vi "SeCrTs-Datalog Redundant NS creater.vi"(9 "Data FIFO Ref":T1, 11 "Queue in":refnum<queue>) -> ()   [LabVIEW 2022 SP3]
uses:
  RT Controls/SeCrTs-Data FIFO.ctl
  RT Controls/SeCrTs-DiplayPC comm ctrl.ctl
  SeCrTs-RT_Global_R.vi
  <resource>/objmgr/ni.dex.rc
panel:
  out "Numeric":i32
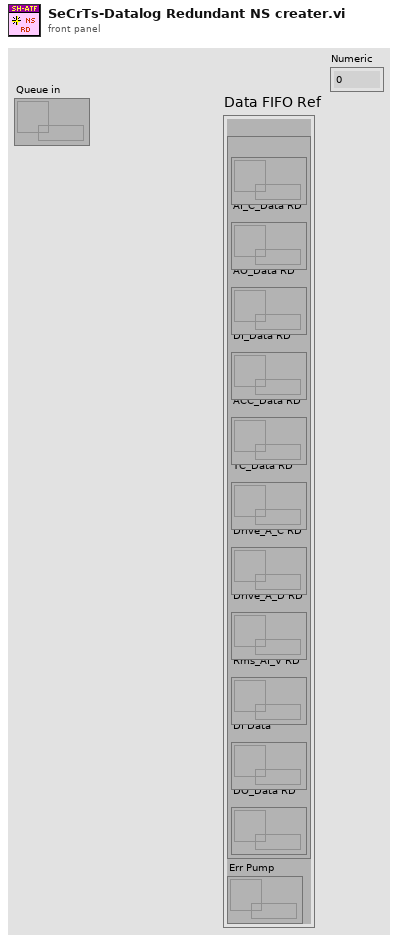
[diagram p1: front panel]
types:
  T1 = typedef "SeCrTs-Data FIFO.ctl" = cluster{"RD":cluster{"AI_V_Data RD":refnum<queue>, "AI_C_Data RD":refnum<queue>, "AO_Data RD":refnum<queue>, "DI_Data RD":refnum<queue>, "ACC_Data RD":refnum<queue>, "TC_Data RD":refnum<queue>, "Drive_A_C RD":refnum<queue>, "Drive_A_D RD":refnum<queue>, "Rms_AI_V RD":refnum<queue>, "DI Data":refnum<queue>, "DO_Data RD":refnum<queue>}, "Err Pump":refnum<queue>}
  T2 = typedef "SeCrTs-DiplayPC comm ctrl.ctl" = enum16{"Initialize", "Listen for UI Writer", "Send RT Data"}
  T3 = cluster{"Start DAQ":bool, "Stop DAQ":bool, "RT Stop":bool, "RT Exit":bool, "Start Seq":bool}
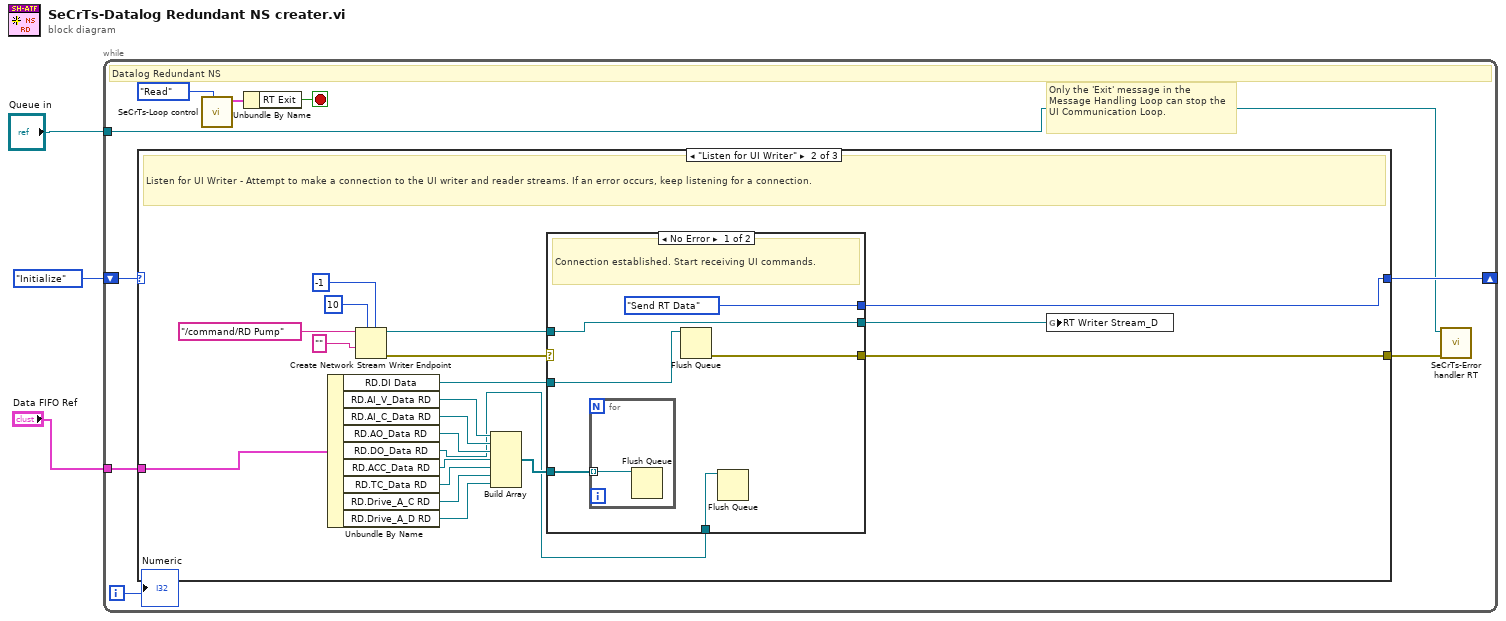
[diagram p0: block diagram]
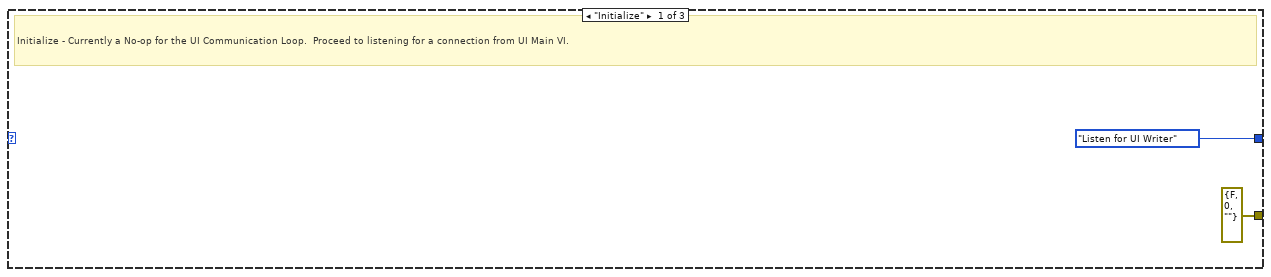
[diagram p2: hidden frame]
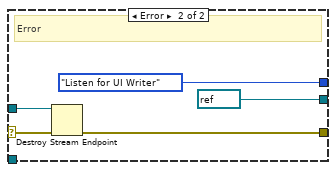
[diagram p3: hidden frame]
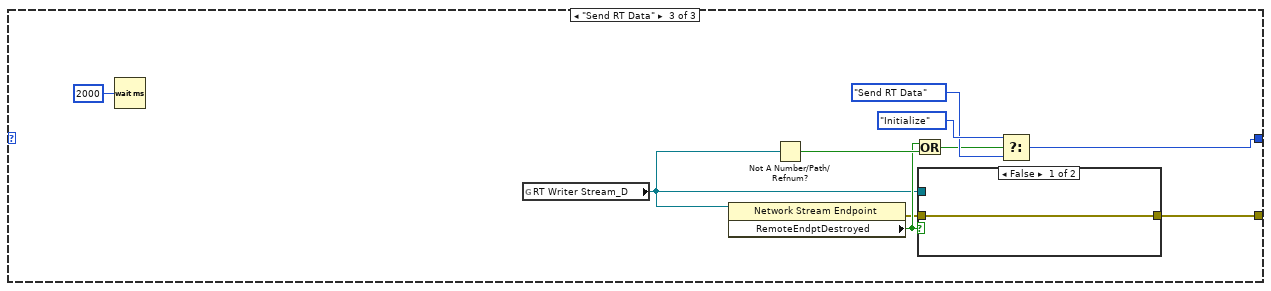
[diagram p4: hidden frame]
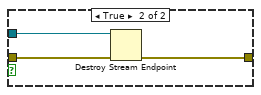
[diagram p5: hidden frame]
diagram:
  n1 = while {
    shift-right: [w12] -> _
    shift-left: SeCrTs-DiplayPC_comm_ctrl."Initialize" -> [w11]
    tunnel: "Data FIFO Ref" -> [w10]
    tunnel: "Queue in" -> [w6]
    i -> [w4]
    stop <- w7 stop-if-true
    # "Only the 'Exit' message in the  Message Handling Loop can stop the UI Communication Loop."
    # "Datalog Redundant NS"
    n2 = case shown="\"Listen for UI Writer\"" w11 {
      tunnel: [errorcluster {"status"=FALSE, "code"=0, "source"=""} ("error IO") w17 w47] -> w5
      tunnel: [SeCrTs-DiplayPC_comm_ctrl."Listen for UI Writer" w32 w54] -> w12
      tunnel: w10 -> [_ w29 _]
      frame "Initialize" {
        # "Initialize - Currently a No-op for the UI Communication Loop.  Proceed to listening for a connection from UI Main VI."
      }
      frame "Listen for UI Writer" {
        # "Listen for UI Writer - Attempt to make a connection to the UI writer and reader streams. If an error occurs, keep listening for a connection."
        n3 = Unbundle By Name(w29) -> ("RD.DI Data"=w18:refnum<queue>, "RD.AI_V_Data RD"=w26:refnum<queue>, "RD.AI_C_Data RD"=w25:refnum<queue>, "RD.AO_Data RD"=w24:refnum<queue>, "RD.DO_Data RD"=w15:refnum<queue>, "RD.ACC_Data RD"=w23:refnum<queue>, "RD.TC_Data RD"=w22:refnum<queue>, "RD.Drive_A_C RD"=w21:refnum<queue>, "RD.Drive_A_D RD"=w20:refnum<queue>)
        n4 = Create Network Stream Writer Endpoint(5:-1 ("timeout in ms (-1)"), 7:10 ("writer buffer size"), 9:"" ("reader url"), 11:"/command/RD Pump" ("reader url")) -> (0:w33:errorcluster, 3:w34:refnum<k21>)  [unwired: 3 in]
        n5 = Build Array(w26, w25, w24, w23, w22, w21, w20) -> (w19:refnum<queue>[])
        n6 = case shown="No Error" w33 {
          selector: w33 -> [_ w44]
          tunnel: w34 -> [w37 w46]
          tunnel: [SeCrTs-DiplayPC_comm_ctrl."Send RT Data" SeCrTs-DiplayPC_comm_ctrl."Listen for UI Writer"] -> w32
          tunnel: [w37 refnum<k21> refnum ("reader url")] -> w27
          tunnel: w19 -> [w39 _]
          tunnel: w18 -> [w38 _]
          tunnel: [w36 w42] -> w17
          tunnel: w15 -> [w35 _]
          frame No Error {
            # "Connection established. Start receiving UI commands."
            n7 = for {
              tunnel: w39 -> [w41] mode=indexing
              n8 = Flush Queue(queue=w41) -> ()  [unwired: 1 in, 3 out]
            }
            n9 = Flush Queue(queue=w38) -> (error out=w36:errorcluster)  [unwired: 1 in, 2 out]
            n10 = Flush Queue(queue=w35) -> ()  [unwired: 1 in, 3 out]
          }
          frame Error {
            # "Error"
            n11 = Destroy Stream Endpoint(8:w44, 11:w46) -> (0:w42:errorcluster)
          }
        }
        n12 = global write "SeCrTs-RT_Global_R.vi" "RT Writer Stream_D"(w27) -> ()
      }
      frame "Send RT Data" {
        n13 = Wait (ms)(milliseconds to wait=u32 2000) -> ()  [unwired: 1 out]
        n14 = global read "SeCrTs-RT_Global_R.vi" "RT Writer Stream_D"() -> (w49:refnum<k21>)
        n15 = property class="Network Stream Endpoint"(reference=w49) -> (error out=w48:errorcluster, "RemoteEndptDestroyed"=w50:bool)  [unwired: 1 in, 1 out]
        n16 = Not A Number/Path/Refnum?(number/path/refnum=w49) -> (NaN/Path/Refnum?=w53:bool)
        n17 = Or(x=w50, y=w53) -> (x .or. y?=w52:bool)
        n18 = case shown="False" w50 {
          tunnel: w49 -> [_ w60]
          tunnel: w48 -> [w57 w59]
          tunnel: [w57 w58] -> w47
          frame False {
          }
          frame True {
            n19 = Destroy Stream Endpoint(8:w59, 11:w60) -> (0:w58:errorcluster)
          }
        }
        n20 = Select(t=SeCrTs-DiplayPC_comm_ctrl."Initialize", s=w52, f=SeCrTs-DiplayPC_comm_ctrl."Send RT Data") -> (s? t:f=w54:T2)
      }
    }
    n21 = call "SeCrTs-Loop control.vi"("Action"=enum16{"Init", "Write", "Read"}."Read") -> ("Loop Control out"=w9:T3)  [unwired: 9 in, 1 out]
    n22 = Unbundle By Name(w9) -> ("RT Exit"=w7:bool)
    n23 = call "SeCrTs-Error handler RT.vi"("error in"=w5, "Message Queue"=w6) -> ()  [unwired: 8 in, 2 out]
    "Numeric" <- w4
  }
